vi "PITSCO myQuake - Basic Example.vi"() -> ()   [LabVIEW 2013]
doc: "A basic example using the myQuake API"
panel:
  out "Acceleration Data":waveform(dbl)[](graph)
  in  "motor output (0%)":dbl(slide) scale=0.0..100.0
  in  "Accelerometer Settings":T1(array[cluster])=[{"Direction"=enum."X - Direction", "Sensitivity"=FALSE}, {"Direction"=enum."X - Direction", "Sensitivity"=FALSE}]
  in  "device name (myDAQ1)":tag="myDAQ1"
  in  "Null Offset":bool
  in  "Stop Button":bool
  # "PITSCO myQuake Example"
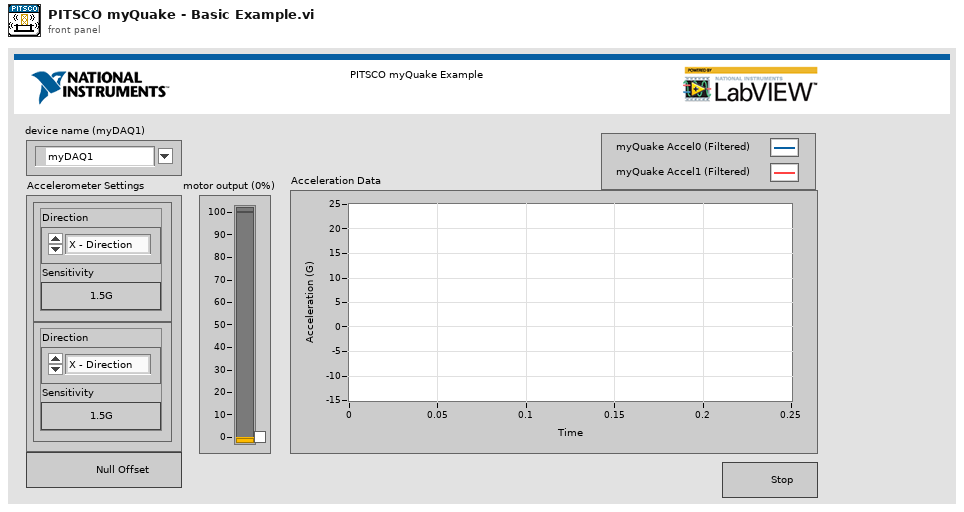
[diagram p1: front panel]
types:
  T1 = cluster{"Direction":enum16{"Off", "X - Direction", "Y - Direction", "Z - Direction"}, "Sensitivity":bool}[]
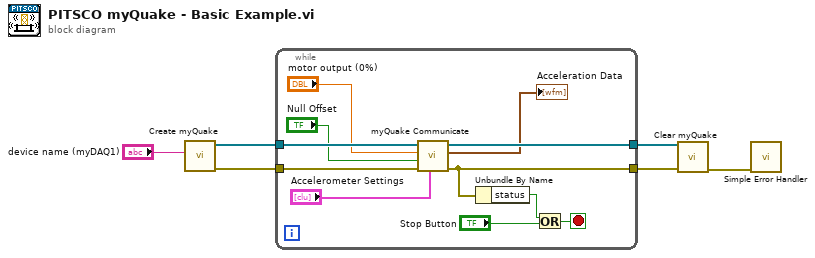
[diagram p0: block diagram]
diagram:
  n1 = call "Create myQuake.vi"("device name (myDAQ1)"="device name (myDAQ1)") -> ("error out"=w5:errorcluster, "task array out"=w6:refnum<k21>[])  [unwired: 8 in, 1 out]
  n2 = while {
    tunnel: w6 -> [w17]
    tunnel: w5 -> [w16]
    tunnel: [w15] -> w3
    tunnel: [w13] -> w4
    stop <- w14 stop-if-true
    n3 = call "myQuake Communicate.vi"("accelerometer settings"="Accelerometer Settings", "error in (no error)"=w16, "set offset (F)"="Null Offset", "motor output (0%)"="motor output (0%)", "task array In"=w17) -> ("error out"=w13:errorcluster, "accel data (g)"=→"Acceleration Data":waveform(dbl)[], "task array out"=w15:refnum<k21>[])  [unwired: 4 in]
    n4 = Unbundle By Name(w13) -> ("status"=w12:bool)
    n5 = Or(x=w12, y="Stop Button") -> (x .or. y?=w14:bool)
  }
  n6 = call "Clear myQuake.vi"("error in (no error)"=w4, "task array In"=w3) -> ("error out"=w2:errorcluster)  [unwired: 9 in]
  n7 = call <vilib>:"Simple Error Handler.vi"("error in (no error)"=w2) -> ()  [unwired: 4 in, 5 out]
